vi "Measurement Logic.vi"() -> ()   [LabVIEW 2020, in "Measurement.lvlib"]
uses:
  Measurement.lvlib
  Measurement Configuration.ctl
  ResolutionInDigits.ctl
  Measurement Results.ctl
  <vilib>/MeasurementLink/MeasurementLink Measurement Server/Measure Call Context/Measure Call Context.lvclass
  <vilib>/MeasurementLink/MeasurementLink Session Management V1/Session Reservation/Initialize and Close Session Behavior.ctl
  FAL/Instrument_Factory/Pin_Instrument_Factory.lvclass
  FAL/Function/Function.lvclass
  <vilib>/MeasurementLink/MeasurementLink Session Management V1/Session Reservation/Session Reservation.lvclass
panel:
  in  "Initialize Behavior":T2
  out "measure call context out":refnum<class "Measure Call Context.lvclass">
  in  "measure call context in":refnum<class "Measure Call Context.lvclass">
  out "measurement results":T3 {"Measurement" format="%.6p"}
  in  "measurement configuration":T4={"pin_name"="", "Range"=10.0, "Measurement Type"=enum."DC Volts", "Resolution in Digits"=enum."5 1/2"} {"Range" format="%.2f"}
  out "error out":errorcluster
  in  "error in":errorcluster
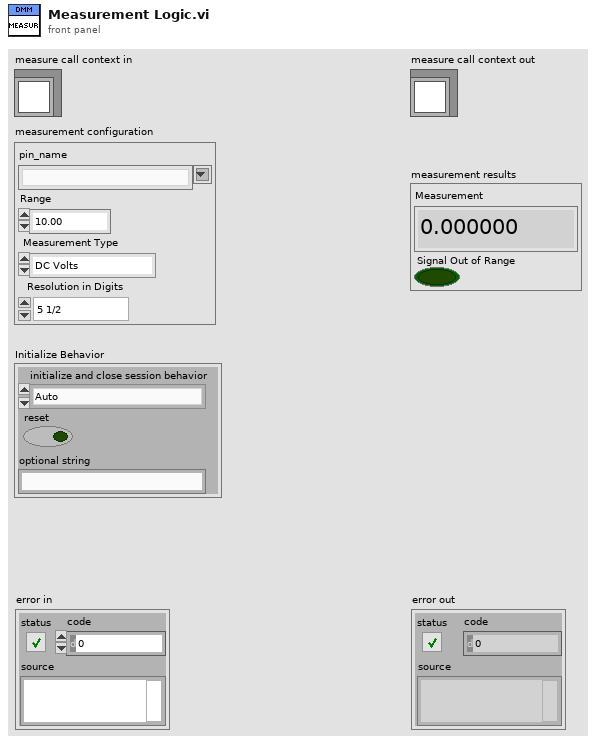
[diagram p1: front panel]
types:
  T1 = typedef "MeasurementLink Session Management V1.lvlib/Session Reservation.lvclass/Initialize and Close Session Behavior.ctl" = enum16{"Auto", "Initialize and Close", "Attach and Detach", "Initialize and Detach", "Attach and Close"}
  T2 = cluster{"initialize and close session behavior":T1, "reset":bool, "optional string":string}
  T3 = typedef "Measurement.lvlib/Measurement Results.ctl" = cluster{"Measurement":dbl, "Signal Out of Range":bool}
  T4 = typedef "Measurement.lvlib/Measurement Configuration.ctl" = cluster{"pin_name":string, "Range":dbl, "Measurement Type":enum32{"DC Volts", "AC Volts", "DC Current", "AC Current", "2-wire Resistance", "4-wire Resistance", "Diode", "Frequency", "Period", "AC Volts DC Coupled", "Capacitance", "Inductance", "Temperature"}, "Resolution in Digits":T5}
  T5 = typedef "Measurement.lvlib/ResolutionInDigits.ctl" = enum32{"3 1/2", "4 1/2", "5 1/2", "6 1/2", "7 1/2"}
  T6 = enum32{"DC Volts", "AC Volts", "DC Current", "AC Current", "2-wire Resistance", "4-wire Resistance", "Diode", "Frequency", "Period", "AC Volts DC Coupled", "Capacitance", "Inductance", "Temperature"}
  T7 = cluster{"session reservation out":refnum<class "Session Reservation.lvclass">, variant[]}
  T8 = cluster{string[], "Range":dbl, "Measurement Type":enum32{"DC Volts", "AC Volts", "DC Current", "AC Current", "2-wire Resistance", "4-wire Resistance", "Diode", "Frequency", "Period", "AC Volts DC Coupled", "Capacitance", "Inductance", "Temperature"}, "Resolution in Digits":T5}
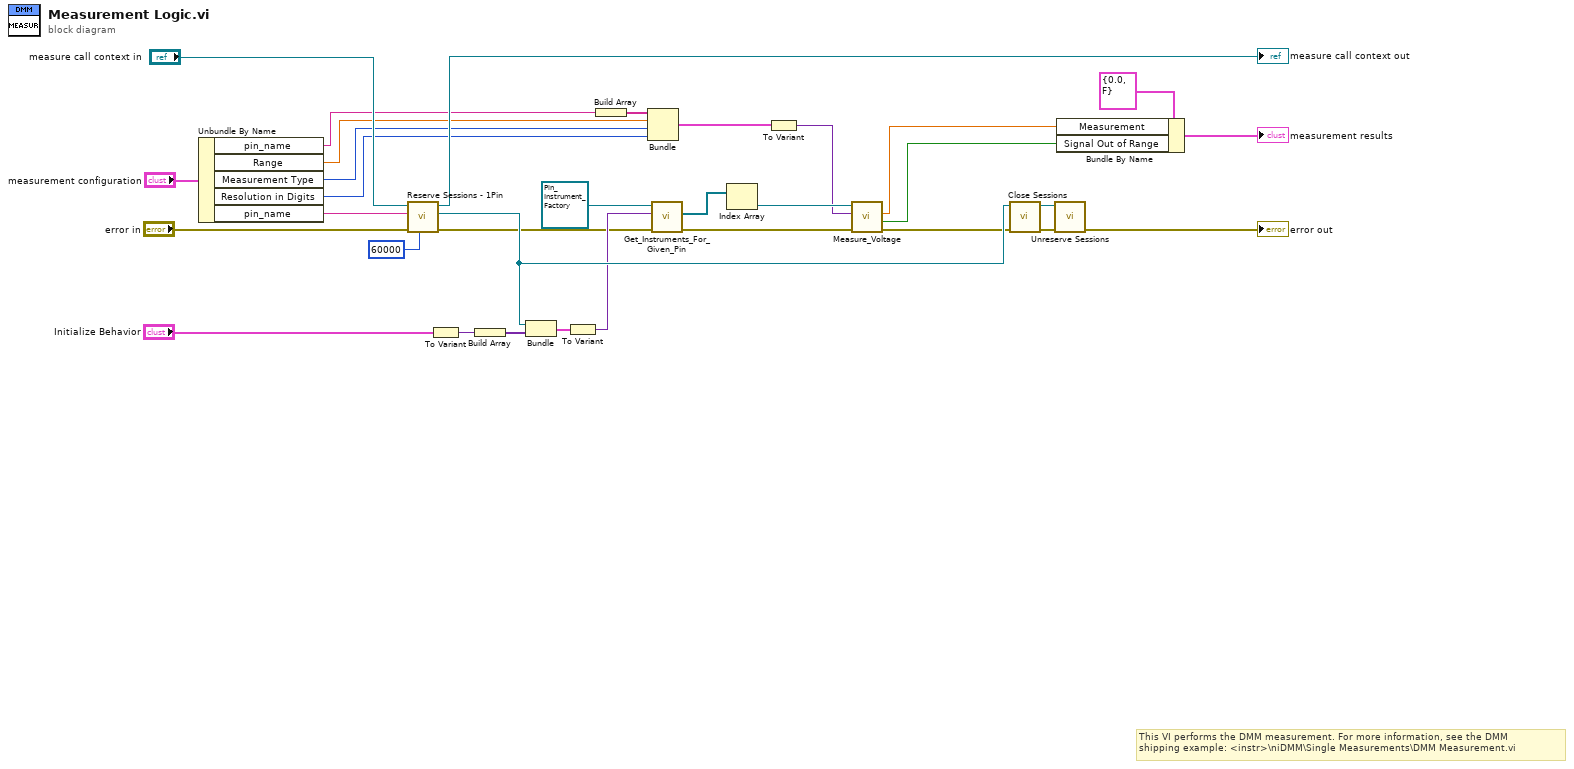
[diagram p0: block diagram]
diagram:
  # "This VI performs the DMM measurement. For more information, see the DMM\nshipping example: <instr>\\niDMM\\Single Measurements\\DMM Measurement.vi"
  n1 = Unbundle By Name("measurement configuration") -> ("pin_name"=w6:string, "Range"=w5:dbl, "Measurement Type"=w4:T6, "Resolution in Digits"=w3:T5, "pin_name"=w8:string)
  n2 = call <vilib>:"Reserve Sessions - 1Pin.vi"("timeout (ms)"=60000, "error in"="error in", "pin or relay name"=w8, "measurement context in"="measure call context in") -> ("error out"=w15:errorcluster, "session reservation out"=w22:refnum<class "Session Reservation.lvclass">, "measurement context out"=→"measure call context out":refnum<class "Measure Call Context.lvclass">)  [unwired: 5 in]
  n3 = To Variant(anything="Initialize Behavior") -> (Variant=w20:variant)
  n4 = Build Array(w20) -> (w19:variant[])
  n5 = Bundle("session reservation out"=w22, w19) -> (w17:T7)  [unwired: 1 in]
  n6 = To Variant(anything=w17) -> (Variant=w18:variant)
  n7 = Build Array(w6) -> (w7:string[])
  n8 = Bundle(w7, "Range"=w5, "Measurement Type"=w4, "Resolution in Digits"=w3) -> (w2:T8)  [unwired: 1 in]
  n9 = call-dynamic "Get_Instruments_For_Given_Pin.vi"("error in (no error)"=w15, "Factory_Data"=w18, "Instrument_Factory in"=refnum<class "Pin_Instrument_Factory.lvclass"> refnum ("Pin_Instrument_Factory.lvclass")) -> ("error out"=w13:errorcluster, "Instrument Functions"=w16:refnum<class "Function.lvclass">[])  [unwired: 6 in, 1 out]
  n10 = Index Array(array=w16) -> (element=w14:refnum<class "Function.lvclass">)  [unwired: 1 in]
  n11 = To Variant(anything=w2) -> (Variant=w9:variant)
  n12 = call-dynamic "Measure_Voltage.vi"("error in"=w13, "Measure_Configuration"=w9, "Function in"=w14) -> ("error out"=w12:errorcluster, "Out of Range"=w1:bool, "DC_Voltage"=w11:dbl)  [unwired: 5 in, 1 out]
  n13 = call <vilib>:"Close Sessions.vi"("error in"=w12, "session reservation in"=w22) -> ("error out"=w30:errorcluster, "session reservation out"=w29:refnum<class "Session Reservation.lvclass">)  [unwired: 8 in]
  n14 = call <vilib>:"Unreserve Sessions.vi"("error in"=w30, "session reservation in"=w29) -> ("error out"=→"error out":errorcluster)  [unwired: 9 in]
  n15 = Bundle By Name(cluster=T3 {"Measurement"=0.0, "Signal Out of Range"=FALSE} ("Measurement Results"), "Measurement"=w11, "Signal Out of Range"=w1) -> (→"measurement results":T3)
